vi "Regional_Weather_Monitoring.vi"() -> ()   [LabVIEW 2018]
uses:
  <vilib>/JDP Science/JSONtext/Find Item.vi
  <vilib>/JDP Science/JSONtext/String Subset.vi
  <vilib>/JDP Science/JSONtext/support/Quote and Escape JSON string.vi
  <vilib>/JDP Science/JSONtext/support/quote and escape json string 2.vi
  <vilib>/JDP Science/JSONtext/Parsing/Parse Full Path or Item Name.vi
  <vilib>/JDP Science/JSONtext/Offset/Find Item Locations by Path.vi
  <vilib>/JDP Science/JSONtext/Offset/Find Object Item Locations by Names.vi
  <vilib>/express/express arith-compare/Formula/XNode/ExpressFormulaBlockNode.xnode
  <vilib>/httpClient/LabVIEWHTTPClient.lvlib
  <vilib>/JDP Science/JSONtext/JSONtext.lvlib
panel:
  out "Slide":u8(slide) scale=0.0..100.0
  out "Wind Direction":dbl(knob) scale=0.0..312.0
  out "Wind Speed(m/s)":dbl(knob) scale=0.0..10.0
  out "Humidity (%)":i32
  out "Humidity Meter":dbl(knob) scale=0.0..100.0
  out "Thermometer":dbl(slide) scale=0.0..50.0
  out "Current Time":timestamp format="%<%I:%M %p\n%x>T"
  out "Sunset (24h)":string
  out "Sunrise (24h)":string
  out "City Chosen":string
  out "Visibility (km)":i32
  out "Wind":T1
  out "Cloud Coverage(%)":cluster{"<JSON>[0]":string}
  out "Status":cluster{"Sky":string, "Description":string}
  out "Pressure (hectoPascal)":string
  in  "Enter City Name":string
  out "Max Temp":dbl
  out "Min Temp":dbl
  out "Feels Like":dbl
  in  "Select °C/°F/K":enum16{"Celcius", "Farenheit", "Kelvin"}(ring)
  out "Current Temp":dbl
  out "Coordinates":cluster{"Longitude":string, "Latitude":string}
  # "Regional Weather Monitoring"
  # "North"
  # "East"
  # "West"
  # "South"
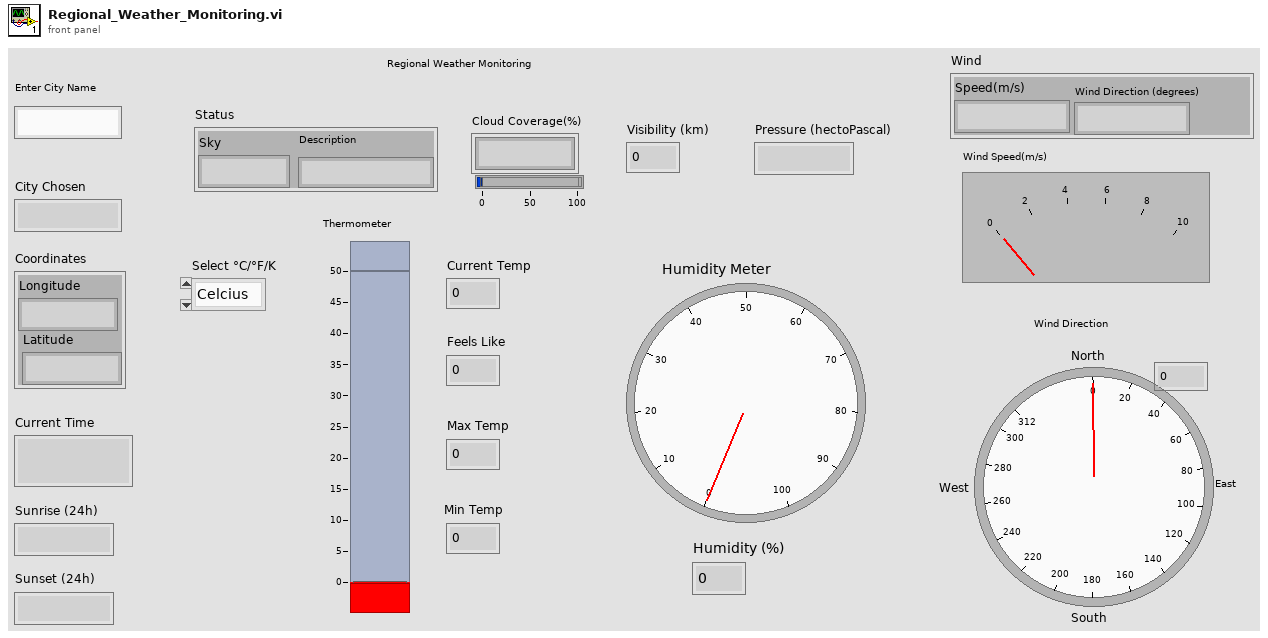
[diagram p1: front panel]
types:
  T1 = cluster{"Speed(m/s)":string, "Wind Direction (degrees)":string}
  T2 = cluster{"<JSON>[0]":string, "<JSON>[1]":string, "<JSON>[2]":string, "<JSON>[3]":string, "<JSON>[4]":string, "<JSON>[5]":string}
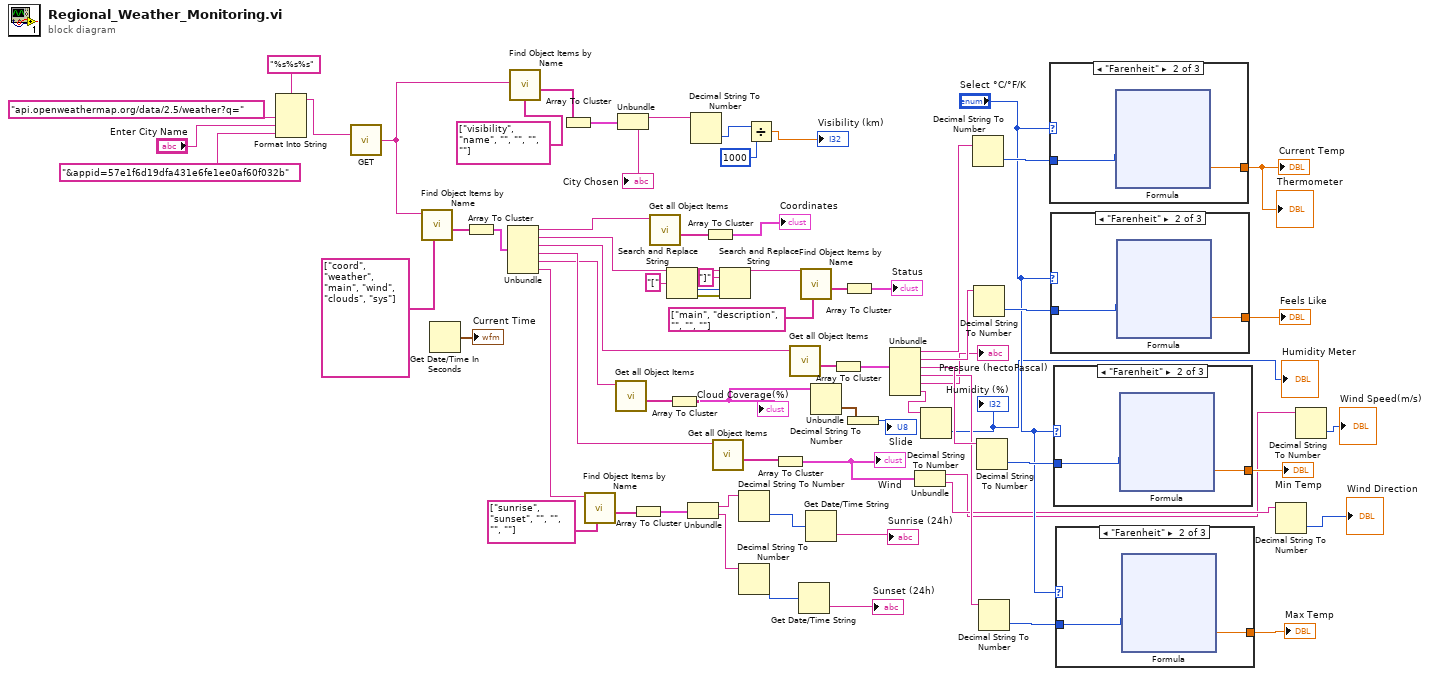
[diagram p0: block diagram]
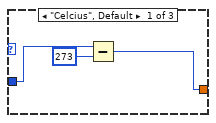
[diagram p2: hidden frame]
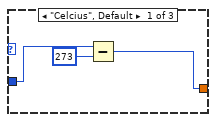
[diagram p4: hidden frame]
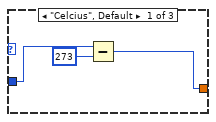
[diagram p6: hidden frame]
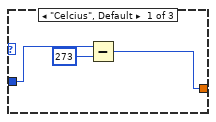
[diagram p8: hidden frame]
diagram:
  n1 = Format Into String "Format Into String"(format string="%s%s%s", "api.openweathermap.org/data/2.5/weather?q=", "Enter City Name", "&appid=57e1f6d19dfa431e6fe1ee0af60f032b" ("url")) -> (resulting string=w39:string)  [unwired: 2 in, 1 out]
  n2 = call <vilib>:"GET.vi"("url"=w39) -> ("body"=w31:string)  [unwired: 11 in, 3 out]
  n3 = call <vilib>:"Find Object Items by Name.vi"("Item Names"=string[] ["coord", "weather", "main", "wind", "clouds", "sys"], "JSON"=w31) -> ("<JSON>"=w71:string[])  [unwired: 7 in, 2 out]
  n4 = Get Date/Time In Seconds() -> (seconds since 1Jan1904=→"Current Time":timestamp)
  n5 = Array To Cluster(array=w71) -> (cluster=w70:T2)
  n6 = Unbundle(w70) -> ("<JSON>[0]"=w69:string, "<JSON>[1]"=w66:string, "<JSON>[2]"=w57:string, "<JSON>[3]"=w34:string, "<JSON>[4]"=w32:string, "<JSON>[5]"=w22:string)
  n7 = call <vilib>:"Find Object Items by Name.vi"("Item Names"=string[] ["visibility", "name", "", "", "", ""], "JSON"=w31) -> ("<JSON>"=w29:string[])  [unwired: 7 in, 2 out]
  n8 = Array To Cluster(array=w29) -> (cluster=w28:cluster{"<JSON>[0]":string, "<JSON>[1]":string})
  n9 = call <vilib>:"Find Object Items by Name.vi"("Item Names"=string[] ["sunrise", "sunset", "", "", "", ""], "JSON"=w22) -> ("<JSON>"=w20:string[])  [unwired: 7 in, 2 out]
  n10 = call <vilib>:"Get all Object Items.vi"("JSON"=w32) -> ("<JSON>"=w37:string[])  [unwired: 7 in, 3 out]
  n11 = Unbundle(w28) -> ("<JSON>[0]"=w27:string, "<JSON>[1]"=→"City Chosen":string)
  n12 = Array To Cluster(array=w20) -> (cluster=w19:cluster{"<JSON>[0]":string, "<JSON>[1]":string})
  n13 = call <vilib>:"Get all Object Items.vi"("JSON"=w69) -> ("<JSON>"=w68:string[])  [unwired: 7 in, 3 out]
  n14 = Search and Replace String(input string=w66, search string="[") -> (result string=w64:string, offset past replacement=w63:i32, error out=w62:errorcluster)  [unwired: 6 in, 1 out]
  n15 = Array To Cluster(array=w37) -> (cluster=w3:cluster{"<JSON>[0]":string})
  "Cloud Coverage(%)" <- w3
  n16 = Unbundle(w19) -> ("<JSON>[0]"=w18:string, "<JSON>[1]"=w13:string)
  n17 = Decimal String To Number(string=w27) -> (number=w26:i32)  [unwired: 2 in, 1 out]
  n18 = Array To Cluster(array=w68) -> (cluster=→"Coordinates":cluster{"<JSON>[0]":string, "<JSON>[1]":string})
  n19 = call <vilib>:"Get all Object Items.vi"("JSON"=w34) -> ("<JSON>"=w33:string[])  [unwired: 7 in, 3 out]
  n20 = Search and Replace String(input string=w64, search string="]", offset=w63, error in=w62) -> (result string=w59:string)  [unwired: 4 in, 3 out]
  n21 = Decimal String To Number(string=w18) -> (number=w17:i32)  [unwired: 2 in, 1 out]
  n22 = Decimal String To Number(string=w13) -> (number=w15:i32)  [unwired: 2 in, 1 out]
  n23 = Divide(x=w26, y=1000) -> (x/y=→"Visibility (km)":dbl)
  n24 = Array To Cluster(array=w33) -> (cluster=w8:cluster{"<JSON>[0]":string, "<JSON>[1]":string})
  "Wind" <- w8
  n25 = call <vilib>:"Get all Object Items.vi"("JSON"=w57) -> ("<JSON>"=w58:string[])  [unwired: 7 in, 3 out]
  n26 = Get Date/Time String(seconds (now)=w15) -> (time string=→"Sunset (24h)":string)  [unwired: 2 in, 1 out]
  n27 = call <vilib>:"Find Object Items by Name.vi"("Item Names"=string[] ["main", "description", "", "", ""], "JSON"=w59) -> ("<JSON>"=w36:string[])  [unwired: 7 in, 2 out]
  n28 = Get Date/Time String(seconds (now)=w17) -> (time string=→"Sunrise (24h)":string)  [unwired: 2 in, 1 out]
  n29 = Decimal String To Number(string=w3) -> (number=w2:cluster{"<JSON>[0]":i32})  [unwired: 2 in, 1 out]
  n30 = Array To Cluster(array=w58) -> (cluster=w56:T2)
  n31 = Array To Cluster(array=w36) -> (cluster=→"Status":cluster{"<JSON>[0]":string, "<JSON>[1]":string})
  n32 = Unbundle(w2) -> ("<JSON>[0]"=→"Slide":i32)
  n33 = Unbundle(w56) -> ("<JSON>[0]"=w55:string, "<JSON>[1]"=w51:string, "<JSON>[2]"=w45:string, "<JSON>[3]"=w44:string, "<JSON>[4]"=→"Pressure (hectoPascal)":string, "<JSON>[5]"=w10:string)
  n34 = Unbundle(w8) -> ("<JSON>[0]"=w5:string, "<JSON>[1]"=w6:string)
  n35 = Decimal String To Number(string=w10) -> (number=→"Humidity Meter" →"Humidity (%)":i32)  [unwired: 2 in, 1 out]
  n36 = Decimal String To Number(string=w55) -> (number=w54:i32)  [unwired: 2 in, 1 out]
  n37 = Decimal String To Number(string=w51) -> (number=w53:i32)  [unwired: 2 in, 1 out]
  n38 = Decimal String To Number(string=w45) -> (number=w50:i32)  [unwired: 2 in, 1 out]
  n39 = Decimal String To Number(string=w44) -> (number=w48:i32)  [unwired: 2 in, 1 out]
  n40 = case shown="\"Farenheit\"" "Select °C/°F/K" {
    tunnel: [w73 w77 w86] -> w11
    tunnel: w54 -> [w75 w76 w86]
    frame "Celcius", Default {
      n41 = Subtract(x=w75, y=273) -> (x-y=w73:i32)
    }
    frame "Farenheit" {
      n42 = xnode "Formula"("X1"=w76) -> ("Result"=w77:dbl)  [unwired: 1 in, 1 out]
    }
    frame "Kelvin" {
    }
  }
  "Current Temp" <- w11
  "Thermometer" <- w11
  n43 = case shown="\"Farenheit\"" "Select °C/°F/K" {
    tunnel: [w87 w91 w100] -> w52
    tunnel: w53 -> [w89 w90 w100]
    frame "Celcius", Default {
      n44 = Subtract(x=w89, y=273) -> (x-y=w87:i32)
    }
    frame "Farenheit" {
      n45 = xnode "Formula"("X1"=w90) -> ("Result"=w91:dbl)  [unwired: 1 in, 1 out]
    }
    frame "Kelvin" {
    }
  }
  "Feels Like" <- w52
  n46 = case shown="\"Farenheit\"" "Select °C/°F/K" {
    tunnel: [w101 w105 w114] -> w49
    tunnel: w50 -> [w103 w104 w114]
    frame "Celcius", Default {
      n47 = Subtract(x=w103, y=273) -> (x-y=w101:i32)
    }
    frame "Farenheit" {
      n48 = xnode "Formula"("X1"=w104) -> ("Result"=w105:dbl)  [unwired: 1 in, 1 out]
    }
    frame "Kelvin" {
    }
  }
  "Min Temp" <- w49
  n49 = case shown="\"Farenheit\"" "Select °C/°F/K" {
    tunnel: [w115 w119 w128] -> w47
    tunnel: w48 -> [w117 w118 w128]
    frame "Celcius", Default {
      n50 = Subtract(x=w117, y=273) -> (x-y=w115:i32)
    }
    frame "Farenheit" {
      n51 = xnode "Formula"("X1"=w118) -> ("Result"=w119:dbl)  [unwired: 1 in, 1 out]
    }
    frame "Kelvin" {
    }
  }
  "Max Temp" <- w47
  n52 = Decimal String To Number(string=w6) -> (number=→"Wind Direction":i32)  [unwired: 2 in, 1 out]
  n53 = Decimal String To Number(string=w5) -> (number=→"Wind Speed(m/s)":i32)  [unwired: 2 in, 1 out]
